vi "发送读取指定ID帧.vi"(0 "T_ID":u32, 5 "R_ID":u32, 7 "CAN_Frame":string, 9 "Time out(ms)":u32=500, 11 "error in (no error)":errorcluster) -> (4 "OK":bool, 6 "Out_Time":bool, 8 "DataLen":u8, 10 "Recive":u8[](array[numeric]), 15 "error out":errorcluster)   [LabVIEW 2020]
uses:
  Libraries/ZLG_CAN/ZLG_CAN.lvlib
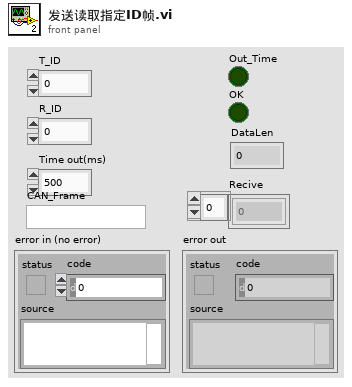
[diagram p1: front panel]
types:
  T1 = typedef "ZLG_CAN.lvlib/CAN_Frame.ctl" = cluster{"[0]":u8, "[1]":u8, "[2]":u8, "[3]":u8, "[4]":u8, "[5]":u8, "[6]":u8, "[7]":u8}
  T2 = typedef "ZLG_CAN.lvlib/Recive_Wait (Reply Payload)--cluster.ctl" = cluster{"Can_Receive":T3[], "Recive_Wait_error":errorcluster}
  T3 = typedef "ZLG_CAN.lvlib/CAN_OBJ_R.ctl" = cluster{"ID":u32, "TimeStamp":u32, "TimeFlag":u8, "SendType":u8, "RemoteFlag":u8, "ExternFlag":u8, "DataLen":u8, "数值":u8, "数值":u8, "数值":u8, "数值":u8, "数值":u8, "数值":u8, "数值":u8, "数值":u8, "数值":u8, "数值":u8, "数值":u8}
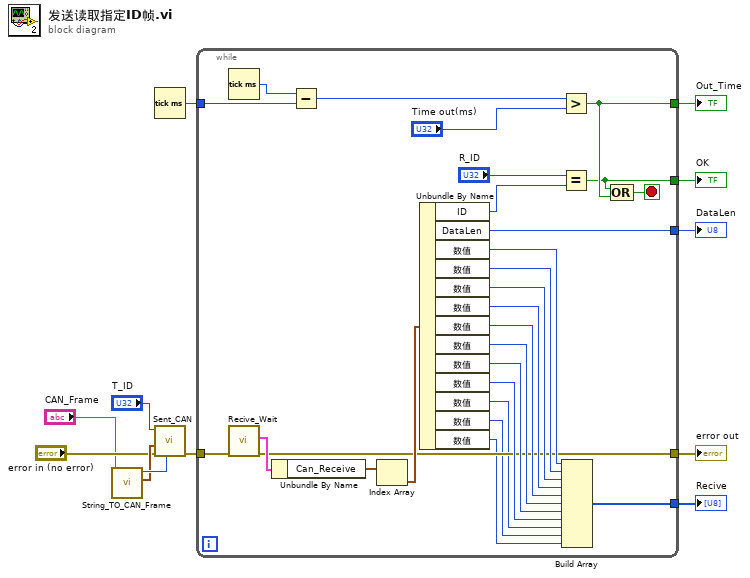
[diagram p0: block diagram]
diagram:
  n1 = call "String_TO_CAN_Frame.vi"("CAN_Frame"="CAN_Frame") -> ("CAN_FRAME"=w11:T1, "DATA_LEN"=w12:i32)  [unwired: 9 in]
  n2 = Tick Count (ms)() -> (millisecond timer value=w6:u32)
  n3 = call "Sent_CAN.vi"("帧长度"=w12, "error in (no error)"="error in (no error)", "帧数据"=w11, "ID"="T_ID") -> ("error out"=w10:errorcluster)  [unwired: 7 in]
  n4 = while {
    tunnel: w10 -> [w37]
    tunnel: [w27] -> w7
    tunnel: w6 -> [w23]
    tunnel: [w20] -> w5
    tunnel: [w15] -> w4
    tunnel: [w14] -> w3
    tunnel: [w13] -> w2
    stop <- w25 stop-if-true
    n5 = Tick Count (ms)() -> (millisecond timer value=w24:u32)
    n6 = call "Recive_Wait.vi"("error in (no error)"=w37) -> ("error out"=w20:errorcluster, "Reply Payload"=w36:T2)  [unwired: 8 in, 1 out]
    n7 = Unbundle By Name(w36) -> ("Can_Receive"=w39:T3[])
    n8 = Subtract(x=w24, y=w23) -> (x-y=w22:u32)
    n9 = Index Array(array=w39) -> (element=w38:T3)  [unwired: 1 in]
    n10 = Unbundle By Name(w38) -> ("ID"=w16:u32, "DataLen"=w15:u8, "数值"=w35:u8, "数值"=w34:u8, "数值"=w33:u8, "数值"=w32:u8, "数值"=w31:u8, "数值"=w30:u8, "数值"=w29:u8, "数值"=w28:u8, "数值"=w19:u8, "数值"=w18:u8, "数值"=w17:u8)
    n11 = Greater?(x=w22, y="Time out(ms)") -> (0:w14:bool)
    n12 = Equal?(x="R_ID", y=w16) -> (x = y?=w13:bool)
    n13 = Build Array(w35, w34, w33, w32, w31, w30, w29, w28, w19, w18, w17) -> (w27:u8[])
    n14 = Compound Arithmetic op=OR ("复合运算")(w13, w14) -> (w25:bool)
  }
  "Recive" <- w7
  "error out" <- w5
  "DataLen" <- w4
  "Out_Time" <- w3
  "OK" <- w2
